vi "Read Fit from File.vi"(8 "error in":errorcluster, 11 "File Path":path) -> (0 "error out":errorcluster, 2 "Fit":dbl[][](array[numeric]))   [LabVIEW 2020]
uses:
  Fit Columns.ctl
panel:
  out "Last index":i32
  out "File data":dbl[](array[numeric])
  in  "Number of columns":dbl
  out "channel name(s) out":string[](array[string])
  out "group name out":string
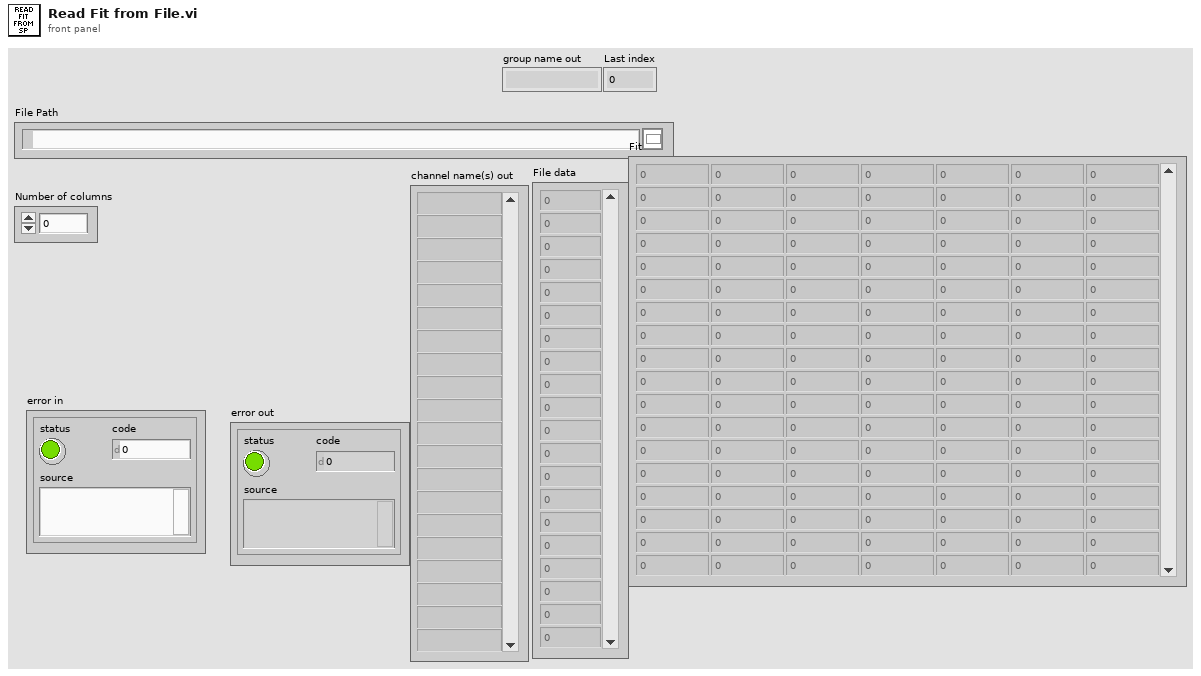
[diagram p1: front panel]
types:
  T1 = typedef "Fit Columns.ctl" = string[]
  T2 = enum16{"open", "open or create", "create or replace", "create", "open (read-only)"}
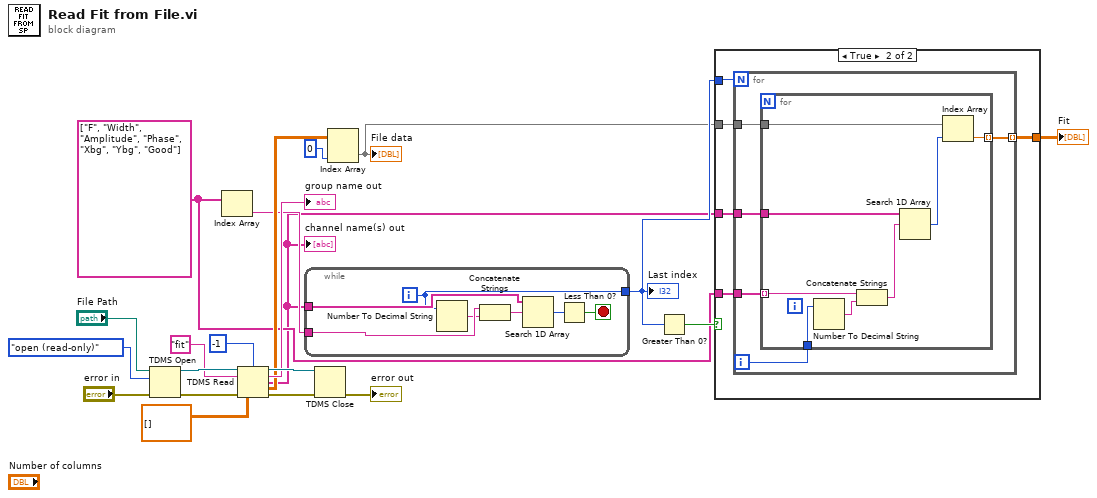
[diagram p0: block diagram]
diagram:
  w4 = T1 ["F", "Width", "Amplitude", "Phase", "Xbg", "Ybg", "Good"] ("Fit columns")
  n1 = TDMS Open(8:"error in", 10:T2."open (read-only)" ("operation (0:open)"), 11:"File Path") -> (0:w18:errorcluster, 3:w17:refnum<k34>)  [unwired: 4 in]
  n2 = Index Array(array=w4) -> (element=w7:string)  [unwired: 1 in]
  n3 = TDMS Read(0:w17, 2:i64 -1 ("count (-1: all)"), 5:"fit" ("group name in"), 11:w18, 12:dbl[][] []) -> (4:w13:refnum<k34>, 6:→"group name out":string, 8:w3:string[], 10:w9:dbl[][], 15:w15:errorcluster)  [unwired: 3 in, 1 out]
  "channel name(s) out" <- w3
  n4 = while {
    tunnel: w7 -> [w28]
    tunnel: w3 -> [w25]
    tunnel: [w22] -> w5
    i -> [w22]
    stop <- w26 stop-if-true
    n5 = Number To Decimal String(number=w22) -> (decimal integer string=w27:string)  [unwired: 1 in]
    n6 = Concatenate Strings(w28, w27) -> (w24:string)
    n7 = Search 1D Array(1D array=w25, element=w24) -> (index of element=w23:i32)  [unwired: 1 in]
    n8 = Less Than 0?(x=w23) -> (x < 0?=w26:bool)
  }
  "Last index" <- w5
  n9 = TDMS Close(8:w15, 11:w13) -> (0:→"error out":errorcluster)  [unwired: 1 out]
  n10 = Index Array(array=w9, index (col)=0 ("index (row)")) -> (element=w2:dbl[])  [unwired: 1 in]
  "File data" <- w2
  n11 = Greater Than 0?(x=w5) -> (x > 0?=w6:bool)
  n12 = case shown="True" w6 {
    tunnel: w5 -> [_ w33]
    tunnel: w4 -> [_ w32]
    tunnel: w3 -> [_ w31]
    tunnel: w2 -> [_ w30]
    tunnel: [_ w29] -> w1
    frame False {
    }
    frame True {
      n13 = for {
        N: w33 -> [_]
        tunnel: w32 -> [w38]
        tunnel: w31 -> [w37]
        tunnel: w30 -> [w36]
        tunnel: [w35] -> w29 mode=indexing
        i -> [w34]
        n14 = for {
          tunnel: w38 -> [w45] mode=indexing
          tunnel: w37 -> [w44]
          tunnel: w36 -> [w42]
          tunnel: [w40] -> w35 mode=indexing
          tunnel: w34 -> [w39]
          n15 = Number To Decimal String(number=w39) -> (decimal integer string=w46:string)  [unwired: 1 in]
          n16 = Concatenate Strings(w45, w46) -> (w43:string)
          n17 = Search 1D Array(1D array=w44, element=w43) -> (index of element=w41:i32)  [unwired: 1 in]
          n18 = Index Array(array=w42, index=w41) -> (element=w40:dbl)
        }
      }
    }
  }
  "Fit" <- w1
